vi "Initialization_Alignment.vi"() -> ()   [LabVIEW 2021]
doc: "André Romero - 2023\nandretec@ifsc.usp.br\nIFSC - USP"
uses:
  Controller.ctl
  Thorlabs-Vector-Move/aptTec/Thorlabs-V2/Global Motors.vi
  Global micro_Devices.vi
panel:
  in  "Tab Control":enum32{"Initialization/Alignment"}(tab)
  in  "step size (mm)":dbl=10.0
  in  "Min   Z":bool
  in  "Max  Z":bool
  in  "Min":bool
  in  "Max":bool
  in  "Z (m/s)":dbl=50.0
  in  "XY (m/s)":dbl format="%#_5g"
  out "Motor Y":bool=TRUE
  out "Motor X":bool=TRUE
  out "Motor Z":bool=TRUE
  in  "Motor - Z":refnum<k7>(container)
  in  "Motor - Y":refnum<k7>(container)
  in  "Motor - X":refnum<k7>(container)
  # "Velocity"
  # "Jog"
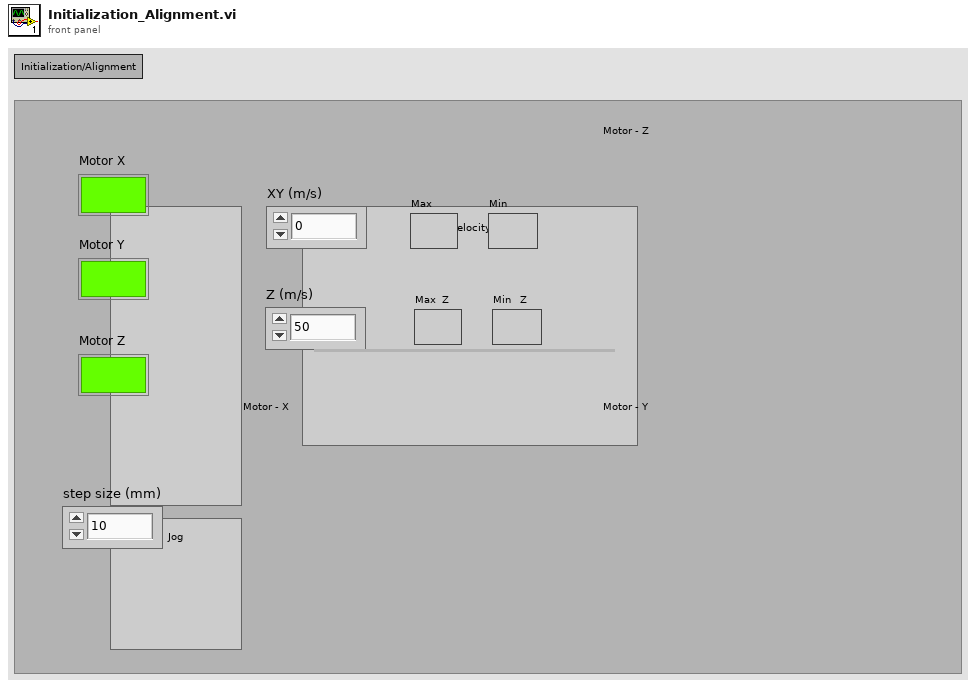
[diagram p1: front panel]
types:
  T1 = typedef "Controller.ctl" = enum16{"Initialize", "Wait for Event", "Cubes", "Lens", "Box", "test tap"}
  T2 = typedef "eventvkey.ctl" = enum16{"ASCII", "Enter", "Return", "Shift", "Ctrl", "Alt", "Cmd", "Opt", "Caps", "NumLock", "Clear", "Break", "Up", "Down", "Left", "Right", "Insert", "Delete", "Home", "End", "PageUp", "PageDown", "Escape", "Help", "Pause", "ScrollLock", "F1", "F2", "F3", "F4", "F5", "F6", "F7", "F8", "F9", "F10", "F11", "F12", "F13", "F14", "F15", "F16", "F17", "F18", "F19", "F20", "F21", "F22", "F23", "F24", "Play", "VolumeUp", "VolumeDown", "Mute", "Two Byte Char"}
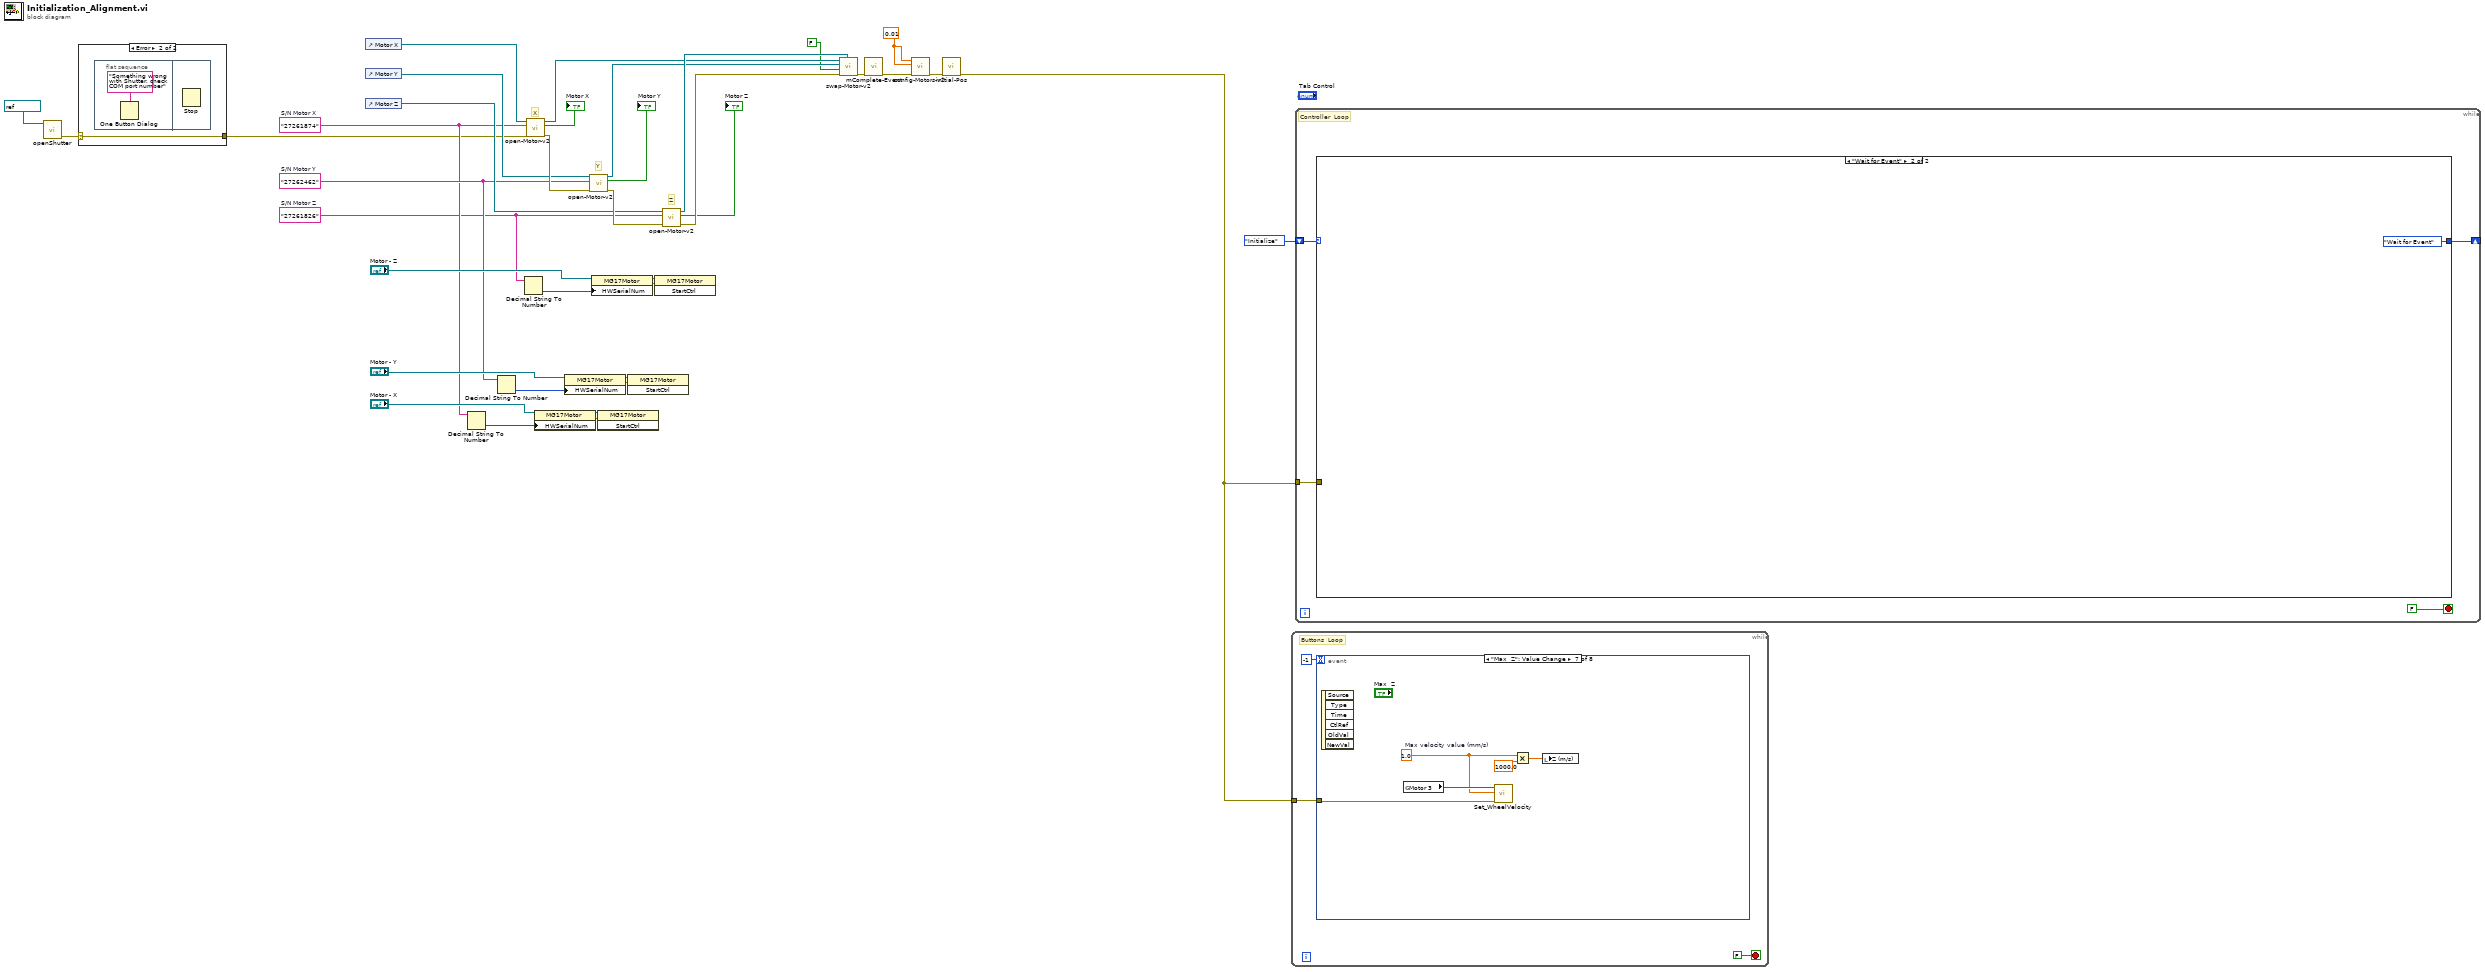
[diagram p0: block diagram]
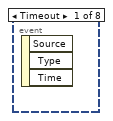
[diagram p3: hidden frame]
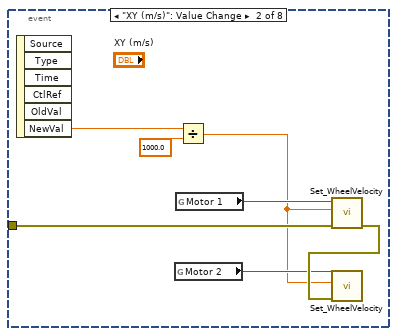
[diagram p4: hidden frame]
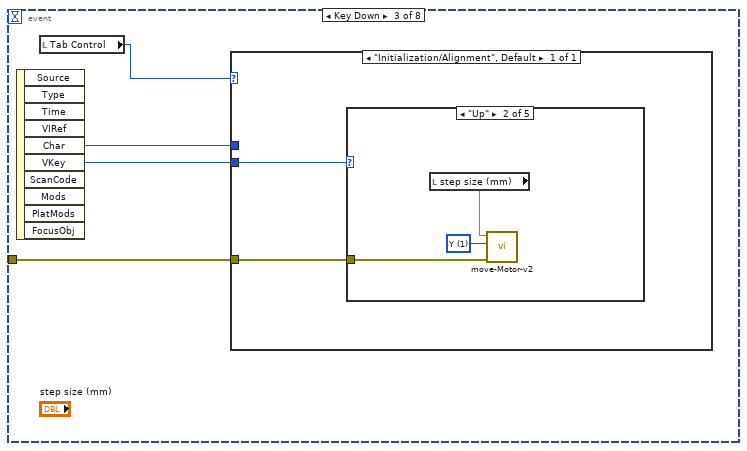
[diagram p5: hidden frame]
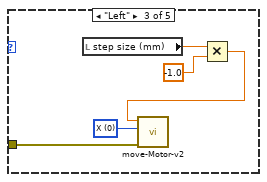
[diagram p7: hidden frame]
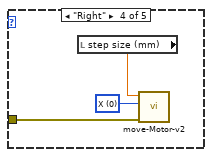
[diagram p8: hidden frame]
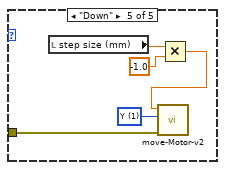
[diagram p9: hidden frame]
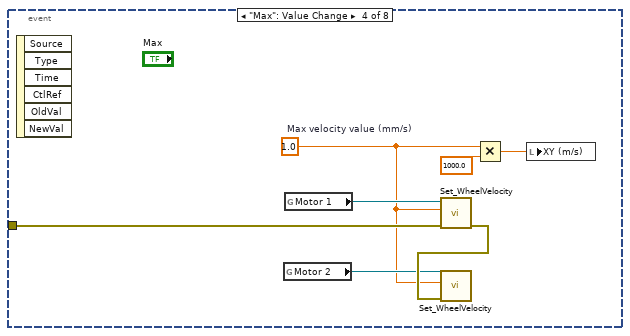
[diagram p10: hidden frame]
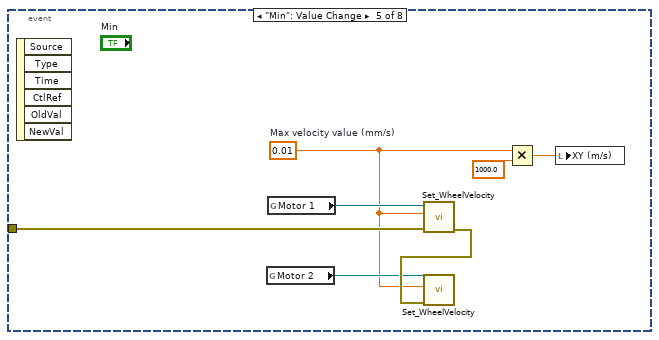
[diagram p11: hidden frame]
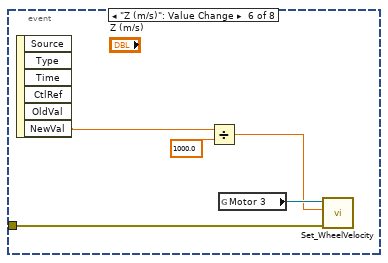
[diagram p12: hidden frame]
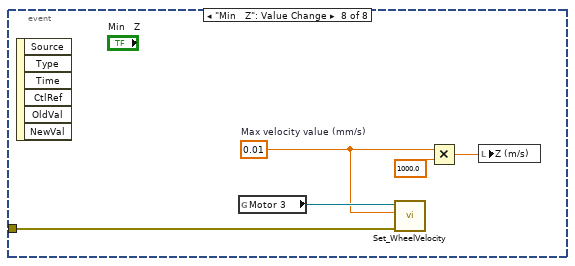
[diagram p13: hidden frame]
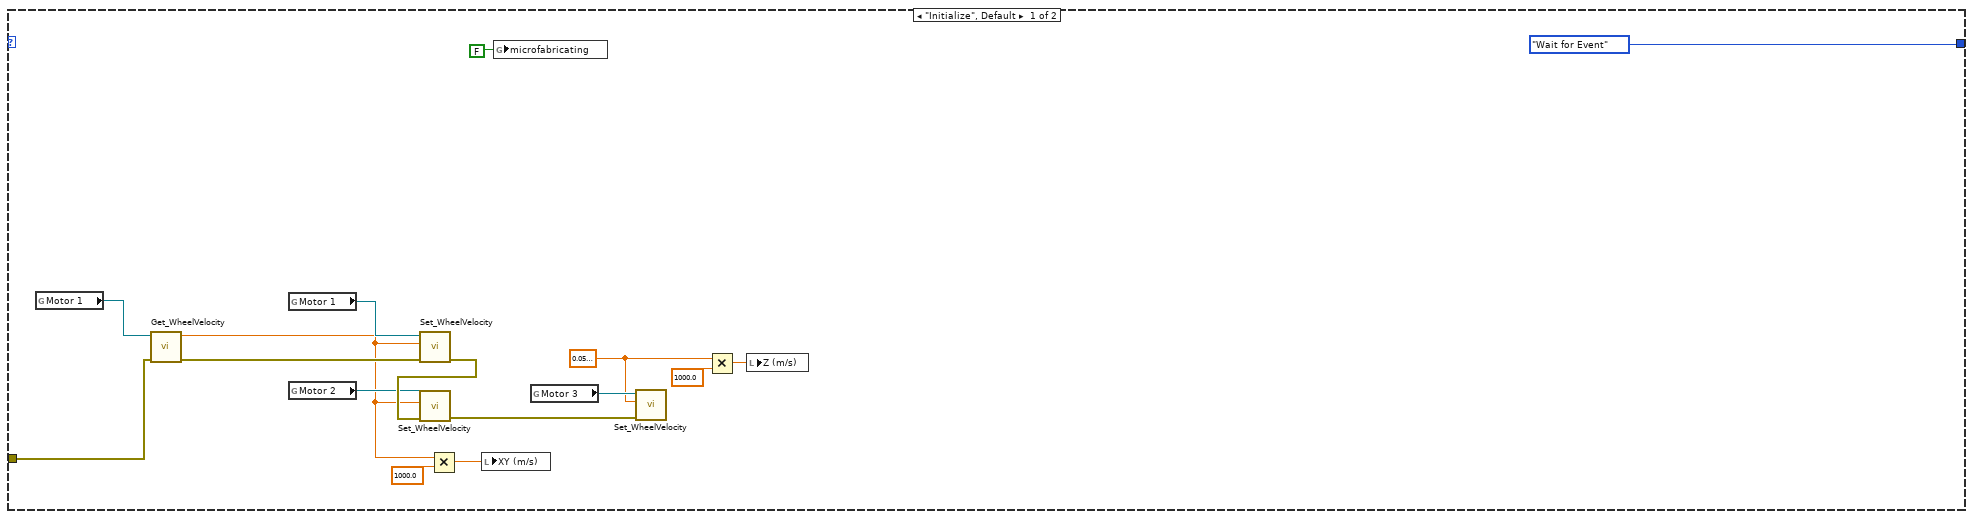
[diagram p14: hidden frame]
diagram:
  w25 = 0.01 ("Acc")
  w12 = "27262462"  # S/N Motor Y
  w11 = "27261874"  # S/N Motor X
  w1 = "27261826"  # S/N Motor Z
  # "X"
  # "Y"
  # "Z"
  n1 = call "openShutter.vi"("VISA Refnum in"=refnum<visa-resource-name> "COM3") -> ("error out"=w3:errorcluster)  [unwired: 9 in, 1 out]
  n2 = case shown="Error" w3 {
    selector: w3 -> [w38 w39]
    tunnel: [w38 w39] -> w2
    frame No Error {
    }
    frame Error {
      n3 = flat-sequence {
        frame #0 {
          n4 = One Button Dialog(message="Something wrong with Shutter, check COM port number") -> ()  [unwired: 1 in, 1 out]
        }
        frame #1 {
          n5 = Stop() -> ()  [unwired: 1 in]
        }
      }
    }
  }
  n6 = control-ref of="Motor X"() -> (w34:refnum<vi>)
  n7 = control-ref of="Motor Y"() -> (w33:refnum<vi>)
  n8 = control-ref of="Motor Z"() -> (w29:refnum<vi>)
  n9 = Decimal String To Number(string=w11) -> (number=w13:i32)  [unwired: 2 in, 1 out]
  n10 = Decimal String To Number(string=w12) -> (number=w17:i32)  [unwired: 2 in, 1 out]
  n11 = Decimal String To Number(string=w1) -> (number=w21:i32)  [unwired: 2 in, 1 out]
  n12 = call "open-Motor-v2.vi"("Error In"=w2, "S/N Motor"=w11, "ref Boolean in"=w34) -> ("Error Out"=w37:errorcluster, "Motor Status"=→"Motor X":bool, "Refnum out"=w7:refnum<k7>)  [unwired: 6 in]
  n13 = property class="MG17Motor"(reference="Motor - X", "HWSerialNum"=w13) -> (reference out=w14:refnum<k7>, error out=w15:errorcluster)  [unwired: 1 in]
  n14 = property class="MG17Motor"(reference="Motor - Y", "HWSerialNum"=w17) -> (reference out=w18:refnum<k7>, error out=w19:errorcluster)  [unwired: 1 in]
  n15 = call "open-Motor-v2.vi"("Error In"=w37, "S/N Motor"=w12, "ref Boolean in"=w33) -> ("Error Out"=w31:errorcluster, "Motor Status"=→"Motor Y":bool, "Refnum out"=w6:refnum<k7>)  [unwired: 6 in]
  n16 = property class="MG17Motor"(reference="Motor - Z", "HWSerialNum"=w21) -> (reference out=w22:refnum<k7>, error out=w23:errorcluster)  [unwired: 1 in]
  n17 = invoke class="MG17Motor" method="StartCtrl"(reference=w14, error in=w15) -> ()  [unwired: 1 in, 3 out]
  n18 = invoke class="MG17Motor" method="StartCtrl"(reference=w18, error in=w19) -> ()  [unwired: 1 in, 3 out]
  n19 = invoke class="MG17Motor" method="StartCtrl"(reference=w22, error in=w23) -> ()  [unwired: 1 in, 3 out]
  n20 = call "open-Motor-v2.vi"("Error In"=w31, "S/N Motor"=w1, "ref Boolean in"=w29) -> ("Error Out"=w30:errorcluster, "Motor Status"=→"Motor Z":bool, "Refnum out"=w27:refnum<k7>)  [unwired: 6 in]
  n21 = call "swap-Motor-v2.vi"("Refnum in M3"=w27, "error in (no error)"=w30, "Swap motor"=FALSE, "Refnum in M2"=w6, "Refnum in M1"=w7) -> ("error out"=w10:errorcluster)  [unwired: 6 in]
  n22 = call "mComplete-Event.vi"("Error In"=w10) -> ("Error Out"=w9:errorcluster)  [unwired: 10 in]
  n23 = call "config-Motors-v2.vi"("error in"=w9, "Acc"=w25, "Velocity"=w25) -> ("error out"=w32:errorcluster)  [unwired: 8 in]
  n24 = call "initial-Pos.vi"("error in (no error)"=w32) -> ("error out"=w8:errorcluster)  [unwired: 10 in]
  n25 = while {
    tunnel: w8 -> [w42]
    stop <- FALSE stop-if-true
    # "Buttons  Loop"
    n26 = event shown="[6] \"Max  Z\": Value Change" {
      selector: _ -> [_ _ _ _ _ _ _ _]
      dyn-events: _ -> [_ _ _ _ _ _ _ _]
      timeout: -1 -> [_ _ _ _ _ _ _ _]
      tunnel: w42 -> [_ w49 w51 w76 w83 w87 w92 w97]
      event Timeout {
        n27 = event-data() -> ()  [unwired: 1 in, 3 out]
      }
      event "XY (m/s)": Value Change {
        n28 = event-data() -> ("NewVal"=w46:dbl)  [unwired: 1 in, 5 out]
        n29 = global read "Global Motors.vi" "Motor 2"() -> (w47:refnum<k7>)
        n30 = global read "Global Motors.vi" "Motor 1"() -> (w50:refnum<k7>)
        n31 = Divide(x=w46, y=1000.0) -> (x/y=w45:dbl)
        n32 = call "Set_WheelVelocity.vi"("error in"=w49, "fWheelVel"=w45, "MG17Motor in"=w50) -> ("error out"=w48:errorcluster)  [unwired: 8 in]
        n33 = call "Set_WheelVelocity.vi"("error in"=w48, "fWheelVel"=w45, "MG17Motor in"=w47) -> ()  [unwired: 8 in, 1 out]
      }
      event Key Down {
        n34 = event-data() -> ("Char"=w53:i16, "VKey"=w52:T2)  [unwired: 1 in, 8 out]
        n35 = local read "Tab Control"() -> (w54:enum32{"Initialization/Alignment"})
        n36 = case shown="\"Initialization/Alignment\", Default" w54 {
          tunnel: w53 -> [_]
          tunnel: w52 -> [w56]
          tunnel: w51 -> [w55]
          frame "Initialization/Alignment", Default {
            n37 = case shown="\"Up\"" w56 {
              tunnel: w55 -> [_ w59 w64 w67 w71]
              frame "ASCII", Default {
              }
              frame "Up" {
                w58 = u16 1 items=["X", "Y", "Z"] ("Axis")
                n38 = local read "step size (mm)"() -> (w57:dbl)
                n39 = call "move-Motor-v2.vi"("error in"=w59, "Axis"=w58, "Distance (um)"=w57) -> ()  [unwired: 8 in, 1 out]
              }
              frame "Left" {
                w63 = u16 0 items=["X", "Y", "Z"] ("Axis")
                n40 = local read "step size (mm)"() -> (w62:dbl)
                n41 = Multiply(x=w62, y=-1.0) -> (x*y=w60:dbl)
                n42 = call "move-Motor-v2.vi"("error in"=w64, "Axis"=w63, "Distance (um)"=w60) -> ()  [unwired: 8 in, 1 out]
              }
              frame "Right" {
                w66 = u16 0 items=["X", "Y", "Z"] ("Axis")
                n43 = local read "step size (mm)"() -> (w65:dbl)
                n44 = call "move-Motor-v2.vi"("error in"=w67, "Axis"=w66, "Distance (um)"=w65) -> ()  [unwired: 8 in, 1 out]
              }
              frame "Down" {
                w72 = u16 1 items=["X", "Y", "Z"] ("Axis")
                n45 = local read "step size (mm)"() -> (w70:dbl)
                n46 = Multiply(x=w70, y=-1.0) -> (x*y=w68:dbl)
                n47 = call "move-Motor-v2.vi"("error in"=w71, "Axis"=w72, "Distance (um)"=w68) -> ()  [unwired: 8 in, 1 out]
              }
            }
          }
        }
      }
      event "Max": Value Change {
        w74 = 1.0  # Max velocity value (mm/s)
        n48 = event-data() -> ()  [unwired: 1 in, 6 out]
        n49 = global read "Global Motors.vi" "Motor 2"() -> (w77:refnum<k7>)
        n50 = global read "Global Motors.vi" "Motor 1"() -> (w79:refnum<k7>)
        n51 = call "Set_WheelVelocity.vi"("error in"=w76, "fWheelVel"=w74, "MG17Motor in"=w79) -> ("error out"=w78:errorcluster)  [unwired: 8 in]
        n52 = call "Set_WheelVelocity.vi"("error in"=w78, "fWheelVel"=w74, "MG17Motor in"=w77) -> ()  [unwired: 8 in, 1 out]
        n53 = Multiply(x=w74, y=1000.0) -> (x*y=w73:dbl)
        n54 = local write "XY (m/s)"(w73) -> ()
      }
      event "Min": Value Change {
        w81 = 0.01  # Max velocity value (mm/s)
        n55 = event-data() -> ()  [unwired: 1 in, 6 out]
        n56 = global read "Global Motors.vi" "Motor 2"() -> (w84:refnum<k7>)
        n57 = global read "Global Motors.vi" "Motor 1"() -> (w86:refnum<k7>)
        n58 = call "Set_WheelVelocity.vi"("error in"=w83, "fWheelVel"=w81, "MG17Motor in"=w86) -> ("error out"=w85:errorcluster)  [unwired: 8 in]
        n59 = call "Set_WheelVelocity.vi"("error in"=w85, "fWheelVel"=w81, "MG17Motor in"=w84) -> ()  [unwired: 8 in, 1 out]
        n60 = Multiply(x=w81, y=1000.0) -> (x*y=w80:dbl)
        n61 = local write "XY (m/s)"(w80) -> ()
      }
      event "Z (m/s)": Value Change {
        n62 = event-data() -> ("NewVal"=w90:dbl)  [unwired: 1 in, 5 out]
        n63 = Divide(x=w90, y=1000.0) -> (x/y=w88:dbl)
        n64 = global read "Global Motors.vi" "Motor 3"() -> (w89:refnum<k7>)
        n65 = call "Set_WheelVelocity.vi"("error in"=w87, "fWheelVel"=w88, "MG17Motor in"=w89) -> ()  [unwired: 8 in, 1 out]
      }
      event "Max  Z": Value Change {
        w94 = 1.0  # Max velocity value (mm/s)
        n66 = event-data() -> ()  [unwired: 1 in, 6 out]
        n67 = global read "Global Motors.vi" "Motor 3"() -> (w96:refnum<k7>)
        n68 = call "Set_WheelVelocity.vi"("error in"=w92, "fWheelVel"=w94, "MG17Motor in"=w96) -> ()  [unwired: 8 in, 1 out]
        n69 = Multiply(x=w94, y=1000.0) -> (x*y=w93:dbl)
        n70 = local write "Z (m/s)"(w93) -> ()
      }
      event "Min   Z": Value Change {
        w99 = 0.01  # Max velocity value (mm/s)
        n71 = event-data() -> ()  [unwired: 1 in, 6 out]
        n72 = global read "Global Motors.vi" "Motor 3"() -> (w101:refnum<k7>)
        n73 = call "Set_WheelVelocity.vi"("error in"=w97, "fWheelVel"=w99, "MG17Motor in"=w101) -> ()  [unwired: 8 in, 1 out]
        n74 = Multiply(x=w99, y=1000.0) -> (x*y=w98:dbl)
        n75 = local write "Z (m/s)"(w98) -> ()
      }
    }
  }
  n76 = while {
    shift-right: [w103] -> _
    shift-left: Controller."Initialize" -> [w104]
    tunnel: w8 -> [w102]
    stop <- FALSE stop-if-true
    # "Controller  Loop"
    n77 = case shown="\"Wait for Event\"" w104 {
      tunnel: [Controller."Wait for Event" Controller."Wait for Event"] -> w103
      tunnel: w102 -> [w106 _]
      frame "Initialize", Default {
        w110 = sgl 0.05 ("fWheelVel")
        n78 = global read "Global Motors.vi" "Motor 1"() -> (w120:refnum<k7>)
        n79 = call "Get_WheelVelocity.vi"("error in"=w106, "MG17Motor in"=w120) -> ("error out"=w116:errorcluster, "pfWheelVel"=w115:sgl)  [unwired: 8 in]
        n80 = global read "Global Motors.vi" "Motor 1"() -> (w119:refnum<k7>)
        n81 = global read "Global Motors.vi" "Motor 2"() -> (w117:refnum<k7>)
        n82 = call "Set_WheelVelocity.vi"("error in"=w116, "fWheelVel"=w115, "MG17Motor in"=w119) -> ("error out"=w118:errorcluster)  [unwired: 8 in]
        n83 = call "Set_WheelVelocity.vi"("error in"=w118, "fWheelVel"=w115, "MG17Motor in"=w117) -> ("error out"=w112:errorcluster)  [unwired: 8 in]
        n84 = Multiply(x=w115, y=sgl 1000.0) -> (x*y=w114:sgl)
        n85 = local write "XY (m/s)"(w114) -> ()
        n86 = global write "Global micro_Devices.vi" "microfabricating"(FALSE ("microfabricating")) -> ()
        n87 = global read "Global Motors.vi" "Motor 3"() -> (w111:refnum<k7>)
        n88 = call "Set_WheelVelocity.vi"("error in"=w112, "fWheelVel"=w110, "MG17Motor in"=w111) -> ()  [unwired: 8 in, 1 out]
        n89 = Multiply(x=w110, y=sgl 1000.0) -> (x*y=w109:sgl)
        n90 = local write "Z (m/s)"(w109) -> ()
      }
      frame "Wait for Event" {
      }
    }
  }
